vi "XML to VI.vi"(6 "VI Path":string, 7 "XML (UTF-8 encoded)":string="<VI _name=\"volume1.vi\">\n  <Control _name=\"radius\" conIdx=\"11\" value=\"T10:0\"/>\n  <Constant outputs=\"four\" value=\"T10:4\"/>\n  <Constant outputs=\"three\" value=\"T10:3\"/>\n  <FixedConst _name=\"PI\" outputs=\"pi\"/>\n  <Multiply inputs=\"radius;radius\" outputs=\"x*y\"/>\n  <Multiply inputs=\"x*y;radius\" outputs=\"x*y2\"/>\n  <Multiply inputs=\"x*y2;four\" outputs=\"x*y3\"/>\n  <Divide inputs=\"x*y3;three\" outputs=\"x/y\"/>\n  <Multiply inputs=\"x/y;pi\" outputs=\"volume\"/>\n  <Indicator _name=\"volume\" conIdx=\"3\" value=\"T10:0\"/>\n</VI>") -> (0 "Error Out":errorcluster)   [LabVIEW 2026]
uses:
  LV AI Core/LV AI Core.lvlib
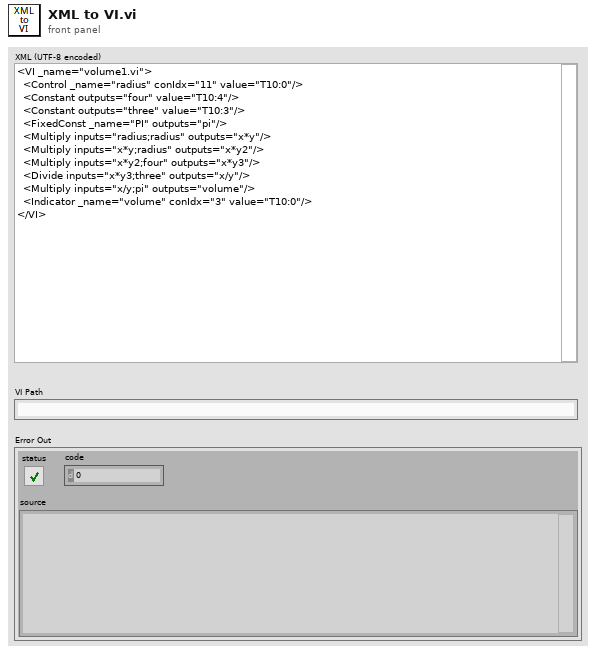
[diagram p1: front panel]
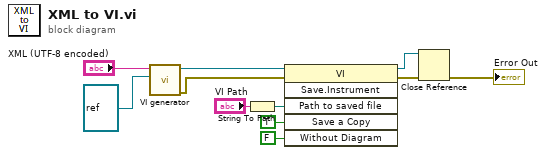
[diagram p0: block diagram]
diagram:
  n1 = call "VI generator.vi"("app ref"=refnum<vi> refnum, "XML (UTF-8 encoded)"="XML (UTF-8 encoded)") -> ("error out"=w3:errorcluster, "vi ref"=w4:refnum<vi>)  [unwired: 8 in]
  n2 = String To Path(string="VI Path") -> (path=w5:path)
  n3 = invoke class="VI" method="Save.Instrument"(reference=w4, error in=w3, "Path to saved file"=w5, "Save a Copy"=TRUE, "Without Diagram"=FALSE) -> (reference out=w9:refnum<vi>, error out=w10:errorcluster)  [unwired: 1 in, 4 out]
  n4 = Close Reference(reference=w9, error in (no error)=w10) -> (error out=→"Error Out":errorcluster)
